vi "Button And Axis To Controller.vi"(6 "All Axis":T15, 7 "Buttons":T14) -> (1 "PS4 Controller":T1={"Square Button"=FALSE, "X Button"=FALSE, "Circle Button"=FALSE, "Triangle Button"=FALSE, "L1"=FALSE, "R1"=FALSE, "Share Button"=FALSE, "Options Button"=FALSE, "PS Button"=FALSE, "Pad Button"=FALSE, "D-Pad"=5, "L2"=0, "R2"=0, "Thumbstick_Left"={[], []}, "Thumbstick_Right"={[], []}} {"R2" scale=-32768.0..32767.0; "L2" scale=-32768.0..32767.0})   [LabVIEW 2020, in "LMH-PS4.lvlib"]
uses:
  LMH-PS4.lvlib
  Type Defs/Axis.ctl
  Type Defs/Indicators/DPad Enum.ctl
  Type Defs/Buttons.ctl
  Type Defs/Indicators/Controller.ctl
  Type Defs/Indicators/Square.ctl
  Type Defs/Indicators/X.ctl
  Type Defs/Indicators/Circle.ctl
  Type Defs/Indicators/Triangle.ctl
  Type Defs/Indicators/L1.ctl
  Type Defs/Indicators/R1.ctl
  Type Defs/Indicators/Share.ctl
  Type Defs/Indicators/Options.ctl
  Type Defs/Indicators/PS.ctl
  Type Defs/Indicators/Pad_Button.ctl
  Type Defs/Indicators/Dpad.ctl
  Type Defs/Indicators/Slider.ctl
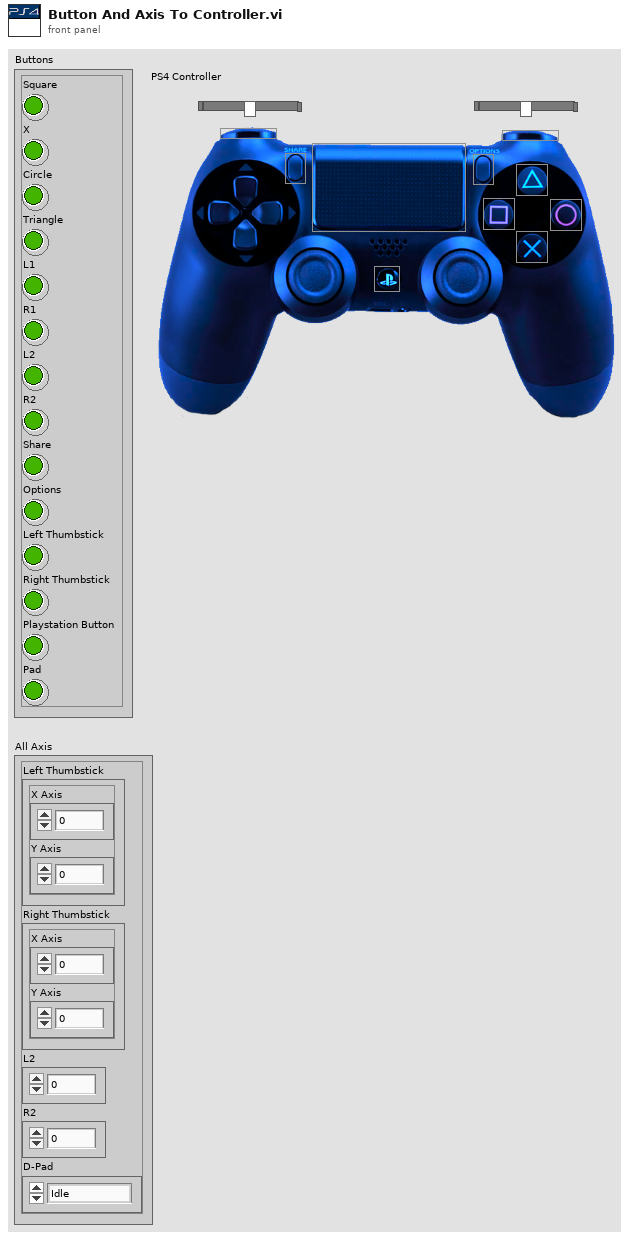
[diagram p1: front panel]
types:
  T1 = typedef "LMH-PS4.lvlib/Controller.ctl" = cluster{"Square Button":T2, "X Button":T3, "Circle Button":T4, "Triangle Button":T5, "L1":T6, "R1":T7, "Share Button":T8, "Options Button":T9, "PS Button":T10, "Pad Button":T11, "D-Pad":T12, "L2":T13, "R2":T13, "Thumbstick_Left":cluster{i32[], i32[]}, "Thumbstick_Right":cluster{i32[], i32[]}}
  T2 = typedef "LMH-PS4.lvlib/Square.ctl" = bool
  T3 = typedef "LMH-PS4.lvlib/X.ctl" = bool
  T4 = typedef "LMH-PS4.lvlib/Circle.ctl" = bool
  T5 = typedef "LMH-PS4.lvlib/Triangle.ctl" = bool
  T6 = typedef "LMH-PS4.lvlib/L1.ctl" = bool
  T7 = typedef "LMH-PS4.lvlib/R1.ctl" = bool
  T8 = typedef "LMH-PS4.lvlib/Share.ctl" = bool
  T9 = typedef "LMH-PS4.lvlib/Options.ctl" = bool
  T10 = typedef "LMH-PS4.lvlib/PS.ctl" = bool
  T11 = typedef "LMH-PS4.lvlib/Pad_Button.ctl" = bool
  T12 = typedef "LMH-PS4.lvlib/Dpad.ctl" = u16
  T13 = typedef "LMH-PS4.lvlib/Slider.ctl" = i32
  T14 = typedef "LMH-PS4.lvlib/Buttons.ctl" = cluster{"Square":bool, "X":bool, "Circle":bool, "Triangle":bool, "L1":bool, "R1":bool, "L2":bool, "R2":bool, "Share":bool, "Options":bool, "Left Thumbstick":bool, "Right Thumbstick":bool, "Playstation Button":bool, "Pad":bool}
  T15 = typedef "LMH-PS4.lvlib/Axis.ctl" = cluster{"Left Thumbstick":cluster{"X Axis":i32, "Y Axis":i32}, "Right Thumbstick":cluster{"X Axis":i32, "Y Axis":i32}, "L2":i32, "R2":i32, "D-Pad":T16}
  T16 = typedef "LMH-PS4.lvlib/DPad Enum.ctl" = enum16{"Idle", "Up", "Up / Right", "Right", "Down / Right", "Down", "Down / Left", "Left", "Up / Left"}
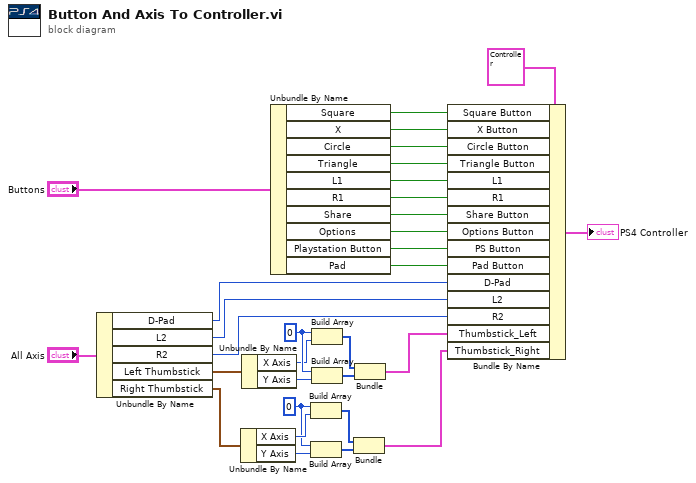
[diagram p0: block diagram]
diagram:
  w21 = 0 ("element")
  w26 = 0 ("element")
  n1 = Unbundle By Name("All Axis") -> ("D-Pad"=w16:T16, "L2"=w15:i32, "R2"=w14:i32, "Left Thumbstick"=w18:cluster{"X Axis":i32, "Y Axis":i32}, "Right Thumbstick"=w17:cluster{"X Axis":i32, "Y Axis":i32})
  n2 = Unbundle By Name(w17) -> ("X Axis"=w22:i32, "Y Axis"=w23:i32)
  n3 = Unbundle By Name(w18) -> ("X Axis"=w25:i32, "Y Axis"=w24:i32)
  n4 = Unbundle By Name("Buttons") -> ("Square"=w11:bool, "X"=w10:bool, "Circle"=w9:bool, "Triangle"=w8:bool, "L1"=w7:bool, "R1"=w6:bool, "Share"=w5:bool, "Options"=w4:bool, "Playstation Button"=w3:bool, "Pad"=w2:bool)
  n5 = Build Array(w21, w22) -> (w19:i32[])
  n6 = Build Array(w21, w23) -> (w20:i32[])
  n7 = Build Array(w26, w25) -> (w28:i32[])
  n8 = Build Array(w26, w24) -> (w27:i32[])
  n9 = Bundle(w19, w20) -> (w12:cluster{i32[], i32[]})  [unwired: 1 in]
  n10 = Bundle(w28, w27) -> (w13:cluster{i32[], i32[]})  [unwired: 1 in]
  n11 = Bundle By Name(cluster=T1 {"Square Button"=FALSE, "X Button"=FALSE, "Circle Button"=FALSE, "Triangle Button"=FALSE, "L1"=FALSE, "R1"=FALSE, "Share Button"=FALSE, "Options Button"=FALSE, "PS Button"=FALSE, "Pad Button"=FALSE, "D-Pad"=5, "L2"=0, "R2"=0, "Thumbstick_Left"={[], []}, "Thumbstick_Right"={[], []}} ("PS4 Controller"), "Square Button"=w11, "X Button"=w10, "Circle Button"=w9, "Triangle Button"=w8, "L1"=w7, "R1"=w6, "Share Button"=w5, "Options Button"=w4, "PS Button"=w3, "Pad Button"=w2, "D-Pad"=w16, "L2"=w15, "R2"=w14, "Thumbstick_Left"=w13, "Thumbstick_Right"=w12) -> (→"PS4 Controller":T1)
